vi "example.vi"() -> ()   [LabVIEW 2010]
panel:
  in  "Some Button":bool
  out "Some Array":dbl[](array[numeric])
  in  "Some String":string
  out "Some Indicator":i32
  in  "Some Control":dbl
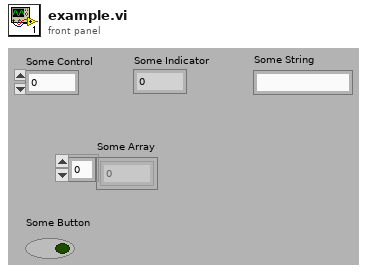
[diagram p1: front panel]
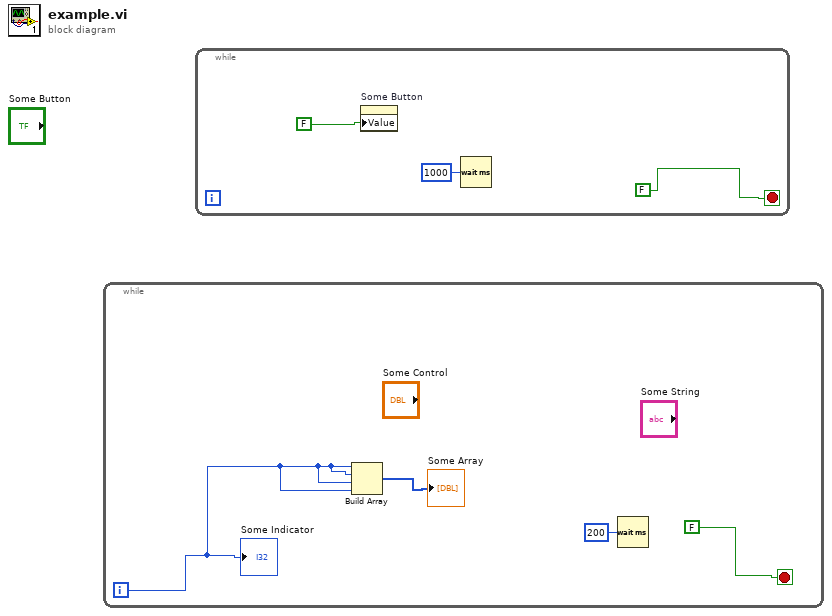
[diagram p0: block diagram]
diagram:
  n1 = while {
    i -> [w3]
    stop <- FALSE ("Some Button") stop-if-true
    n2 = Build Array(w3, w3, w3, w3) -> (→"Some Array":i32[])
    n3 = Wait (ms)(milliseconds to wait=u32 200) -> ()  [unwired: 1 out]
    "Some Indicator" <- w3
  }
  n4 = while {
    stop <- FALSE ("Some Button") stop-if-true
    n5 = property on="Some Button" class="Bool (strict)"("Value"=FALSE ("Some Button")) -> ()  [unwired: 2 in, 2 out]
    n6 = Wait (ms)(milliseconds to wait=u32 1000) -> ()  [unwired: 1 out]
  }
